vi "TSM SSC DCPower Pins to Sessions.vi"(0 "TSM context":T6, 1 "Fill SSC Pin and Site Information? (T)":bool=TRUE, 5 "Pins":tag[](array[tag]), 7 "Site Numbers":i32[](array[numeric]), 11 "error in":errorcluster) -> (4 "DCPower TSM Out":T1, 15 "error out":errorcluster)   [LabVIEW 2019]
doc: "Populates the TSM SSC DCPower cluster for the specified pin(s) and pin group(s). \n\nThe \"Fill SSC Pin and Site Information?\" should be set to TRUE (the default value) so the DCPower SSC cluster has full information about what DCPower sessions correspond to what DUT Pins. This assists in debugging and allows for correlating arrays back to the original list of pins provided to pins to sessions.\n\nThe \"Fill SSC Pin and Site Information?\" input can be set to FALSE if these features aren't needed, or to optimize test time."
uses:
  <vilib>/NI_TestStand_SemiconductorModule/NI_TestStand_Semiconductor_Module.lvlibp/PinMap/General/SemiconductorModuleContext.ctl
  TSM SSC DCPower.ctl
  <vilib>/NI_TestStand_SemiconductorModule/NI_TestStand_Semiconductor_Module.lvlibp/PinMap/PinQueryContext/MultiplePinMultipleSessionQueryContext/MultiplePinMultipleSessionQueryContext.lvclass
  C:/Program Files/National Instruments/LabVIEW 2019/vi.lib/NI_TestStand_SemiconductorModule/NI_TestStand_Semiconductor_Module.lvlibp/PinMap/PinQueryContext/PinQueryContext.lvclass
  SSC DCPower/SSC DCPower.ctl
  Shared SubVIs/TSM Pin Abstraction/TSM Pin Information.ctl
  Shared SubVIs/TSM Pin Abstraction/TSM Pin Type Identifier.ctl
  Shared SubVIs/TSM Pin Abstraction/TSM Expanded Pin Information.ctl
  <vilib>/NI_TestStand_SemiconductorModule/NI_TestStand_Semiconductor_Module.lvlibp/PinMap/DC Power/PinsToNIDCPowerSessions.vi
  <vilib>/NI_TestStand_SemiconductorModule/NI_TestStand_Semiconductor_Module.lvlibp
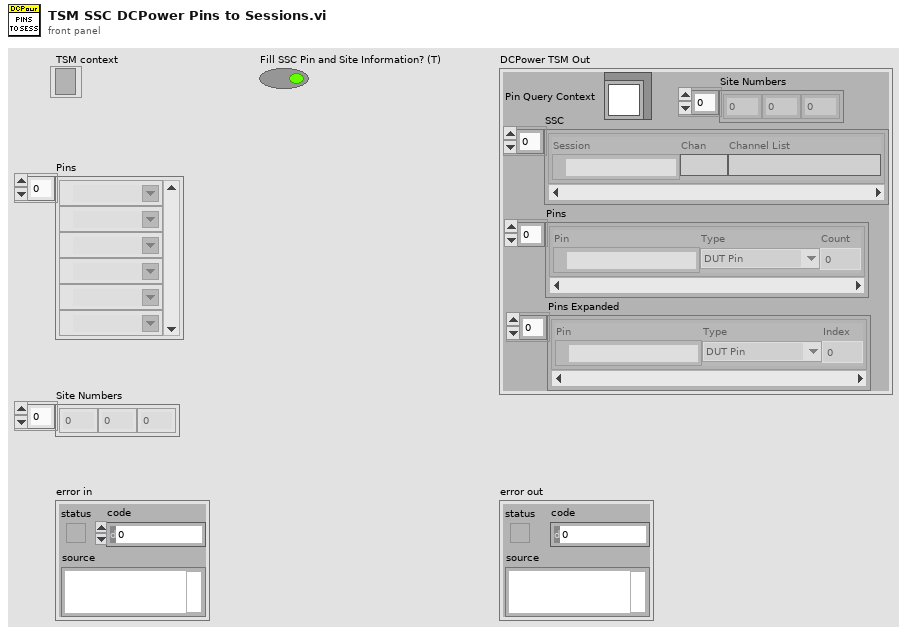
[diagram p1: front panel]
types:
  T1 = typedef "TSM SSC DCPower.ctl" = cluster{"Pin Query Context":refnum<class "MultiplePinMultipleSessionQueryContext.lvclass">, "SSC":T2[], "Site Numbers":i32[], "Pins":T3[], "Pins Expanded":T5[]}
  T2 = typedef "SSC DCPower.ctl" = cluster{"Session":refnum<k15>, "Chan":string, "Channel List":string}
  T3 = typedef "TSM Pin Information.ctl" = cluster{"Pin":tag, "Type":T4, "Count":i32}
  T4 = typedef "TSM Pin Type Identifier.ctl" = enum8{"DUT Pin", "System Pin", "Pin Group", "Not Determined"}
  T5 = typedef "TSM Expanded Pin Information.ctl" = cluster{"Pin":tag, "Type":T4, "Index":i32}
  T6 = typedef "NI_TestStand_Semiconductor_Module.lvlibp/SemiconductorModuleContext.ctl" = refnum<k7>
  T7 = cluster{"Instrument Session":refnum<k15>, "Channel List":string, "spreadsheet string":string}[]
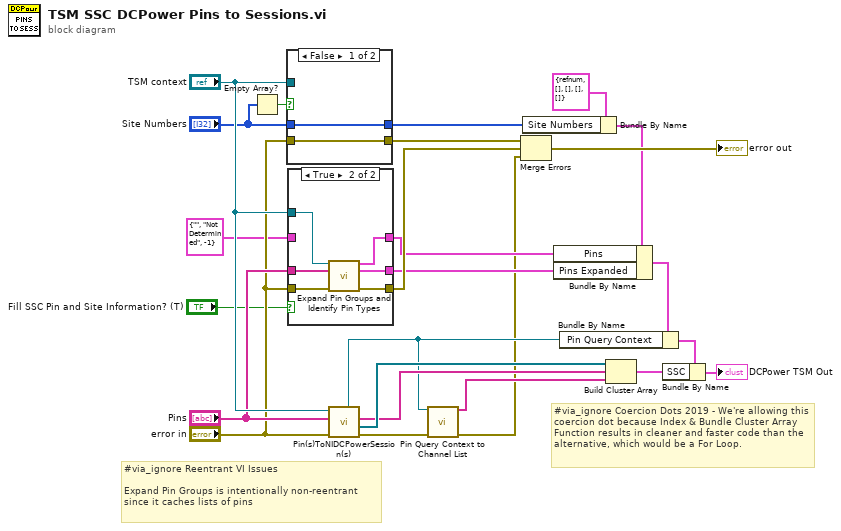
[diagram p0: block diagram]
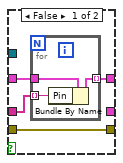
[diagram p2: hidden frame]
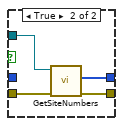
[diagram p3: hidden frame]
diagram:
  # "#via_ignore Reentrant VI Issues\n\nExpand Pin Groups is intentionally non-reentrant\nsince it caches lists of pins"
  # "#via_ignore Coercion Dots 2019 - We're allowing this coercion dot because Index & Bundle Cluster Array Function results in cleaner and faster code than the alternative, which would be a For Loop."
  n1 = Empty Array?(array="Site Numbers") -> (empty?=w19:bool)
  n2 = case shown="False" w19 {
    tunnel: "error in" -> [w26 w31]
    tunnel: [w26 w30] -> w15
    tunnel: "TSM context" -> [_ w29]
    tunnel: [w27 w28] -> w5
    tunnel: "Site Numbers" -> [w27 _]
    frame False {
    }
    frame True {
      n3 = call <vilib>:"GetSiteNumbers.vi"("error in (no error)"=w31, "Semiconductor Module Context"=w29) -> ("error out"=w30:errorcluster, "Site Numbers"=w28:i32[])  [unwired: 6 in, 2 out]
    }
  }
  n4 = case shown="True" "Fill SSC Pin and Site Information? (T)" {
    tunnel: "TSM context" -> [_ w44]
    tunnel: "Pins" -> [w33 w43]
    tunnel: "error in" -> [w35 w42]
    tunnel: [w35 w41] -> w14
    tunnel: [w32 w40] -> w10
    tunnel: [_ w39] -> w6
    tunnel: T3 {"Pin"="", "Type"=enum."Not Determined", "Count"=-1} ("Pin Information") -> [w34 _]
    frame False {
      n5 = for {
        tunnel: w34 -> [w38]
        tunnel: w33 -> [w37] mode=indexing
        tunnel: [w36] -> w32 mode=indexing
        n6 = Bundle By Name(cluster=w38, "Pin"=w37) -> (w36:T3)
      }
    }
    frame True {
      n7 = call "Expand Pin Groups and Identify Pin Types.vi"("TSM context"=w44, "Pins and/or Pin Groups"=w43, "error in"=w42) -> ("Pins and/or Pin Groups Information"=w40:T3[], "Expanded Pin Information"=w39:T5[], "error out"=w41:errorcluster)  [unwired: 10 in]
    }
  }
  n8 = call-poly <vilib>:"Pin(s)ToNIDCPowerSession(s).vi"("error in (no error)"="error in", "Pins"="Pins", "Semiconductor Module Context"="TSM context") -> ("error out"=w3:errorcluster, "Instrument Sessions"=w25:refnum<k15>[], "Channel Lists"=w24:string[], "Pin Query Context"=w4:refnum<class "MultiplePinMultipleSessionQueryContext.lvclass">)  [unwired: 4 in, 1 out]
  n9 = call "Pin Query Context to Channel List.vi"("Pin Query Context"=w4, "error in"=w3) -> ("Per-Session Channel List"=w2:string[], "error out"=w1:errorcluster)  [unwired: 11 in, 1 out]
  n10 = Merge Errors(w15, w14, w1) -> (→"error out":errorcluster)
  n11 = Bundle By Name(cluster=T1 {"Pin Query Context"=refnum, "SSC"=[], "Site Numbers"=[], "Pins"=[], "Pins Expanded"=[]} ("DAQmx - Multiple Sessions Info"), "Site Numbers"=w5) -> (w12:T1)
  n12 = Bundle By Name(cluster=w12, "Pins"=w10, "Pins Expanded"=w6) -> (w11:T1)
  n13 = Bundle By Name(cluster=w11, "Pin Query Context"=w4) -> (w9:T1)
  n14 = Build Cluster Array(w25, w24, w2) -> (w22:T7)
  n15 = Bundle By Name(cluster=w9, "SSC"=w22) -> (→"DCPower TSM Out":T1)
